vi "Channel Cluster to Table.vi"(11 "channel settings":T1) -> (3 "channel settings table":string[][](table))   [LabVIEW 2020, in "Ballard MIL-STD-1553 System Explorer.lvlib" / "Implementation.lvlib"]
uses:
  Implementation.lvlib
  <vilib>/NI VeriStand/Custom Device API/Custom Device Channel.ctl
  <vilib>/NI VeriStand/Custom Device API/Custom Device Channel Type.ctl
  <vilib>/NI VeriStand/Custom Device API/Custom Device API.lvlib
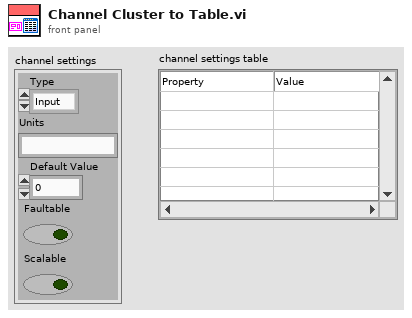
[diagram p1: front panel]
types:
  T1 = typedef "Custom Device API.lvlib/Custom Device Channel.ctl" = cluster{"Type":T2, "Units":string, "Default Value":dbl, "Faultable":bool, "Scalable":bool}
  T2 = typedef "Custom Device API.lvlib/Custom Device Channel Type.ctl" = enum16{"Input", "Output"}
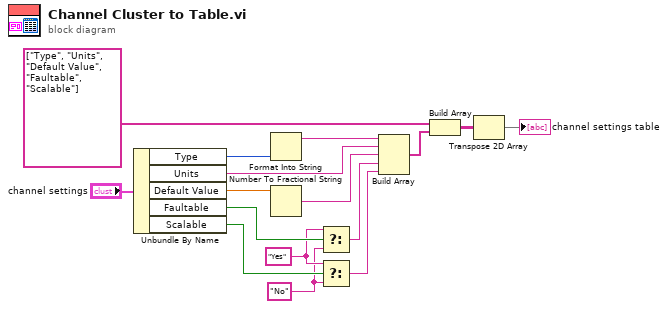
[diagram p0: block diagram]
diagram:
  w7 = "No"
  w8 = "Yes"
  n1 = Unbundle By Name("channel settings") -> ("Type"=w6:T2, "Units"=w13:string, "Default Value"=w5:dbl, "Faultable"=w11:bool, "Scalable"=w15:bool)
  n2 = Format Into String(w6) -> (resulting string=w14:string)  [unwired: 3 in, 1 out]
  n3 = Number To Fractional String(number=w5) -> (F-format string=w12:string)  [unwired: 3 in]
  n4 = Select(t=w8, s=w11, f=w7) -> (s? t:f=w10:string)
  n5 = Select(t=w8, s=w15, f=w7) -> (s? t:f=w9:string)
  n6 = Build Array(w14, w13, w12, w10, w9) -> (w4:string[])
  n7 = Build Array(string[] ["Type", "Units", "Default Value", "Faultable", "Scalable"] ("channel settings table"), w4) -> (w2:string[][])
  n8 = Transpose 2D Array(2D array=w2) -> (transposed array=→"channel settings table":string[][])
